vi "Y4(t).vi"(1 "Initial Position":dbl, 2 "L":dbl, 3 "W":dbl, 4 "V":dbl, 5 "T":dbl) -> (0 "Y4(t)":dbl)   [LabVIEW 2012]
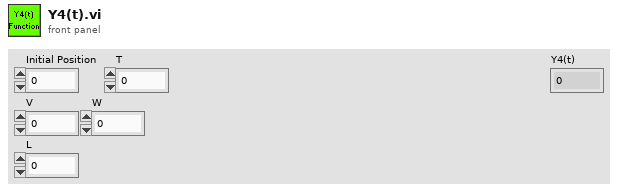
[diagram p1: front panel]
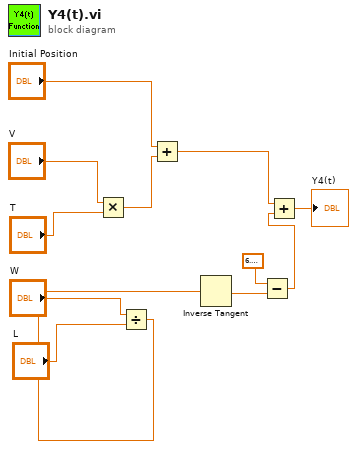
[diagram p0: block diagram]
diagram:
  n1 = Multiply(x="V", y="T") -> (x*y=w10:dbl)
  n2 = Divide(x="W", y="L") -> (x/y=w6:dbl)
  n3 = Add(x="Initial Position", y=w10) -> (x+y=w2:dbl)
  n4 = Inverse Tangent(1:w6) -> (0:w5:dbl)
  n5 = Subtract(x=6.283185307179586, y=w5) -> (x-y=w3:dbl)
  n6 = Add(x=w2, y=w3) -> (x+y=→"Y4(t)":dbl)
